vi "SVI_gauss_proba.vi"(4 "Delta":dbl, 5 "Seuil":dbl) -> (0 "Mu+ Delta":dbl, 1 "Mu-Delta":dbl, 2 "proba (Mu-Delta<X< Mu + Delta)":dbl(knob) scale=0.0..100.0, 3 "proba (X<Seuil)":dbl(knob) scale=0.0..100.0)   [LabVIEW 2010, in "lv_02.lvlib"]
uses:
  lv_02/p_5E1_LN.ctl
  lv_02/lv_02.lvlib
panel:
  in  "Paramètres Loi de Gauss":T1
  # "MODELE DE GAUSS\nF(Seuil)=prob(X<Seuil) \nprob (m-Delta<X<m+delta) \nsi X ---> N(m,sigma)"
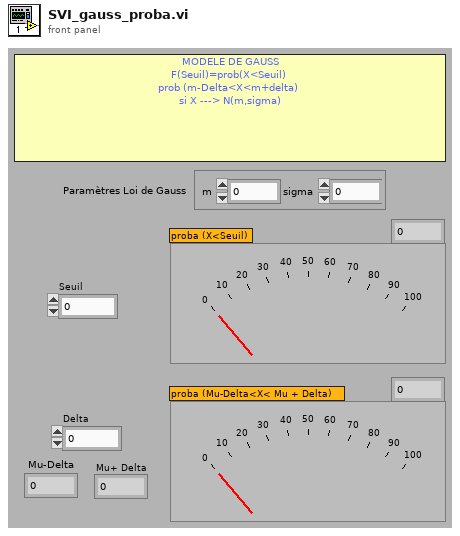
[diagram p1: front panel]
types:
  T1 = typedef "lv_02.lvlib/p_5E1_LN.ctl" = cluster{"m":dbl, "sigma":dbl}
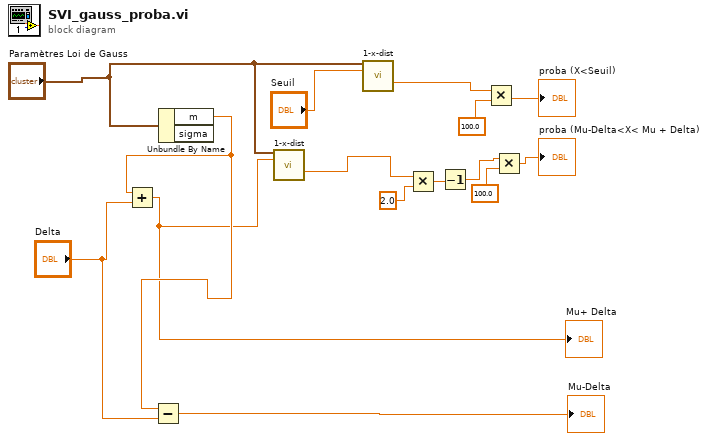
[diagram p0: block diagram]
diagram:
  n1 = Unbundle By Name("Paramètres Loi de Gauss") -> ("m"=w4:dbl)  [unwired: 1 out]
  n2 = Add(x=w4, y="Delta") -> (x+y=w2:dbl)
  "Mu+ Delta" <- w2
  n3 = Subtract(x=w4, y="Delta") -> (x-y=→"Mu-Delta":dbl)
  n4 = call "1-x-dist.vi"("p_LN"="Paramètres Loi de Gauss", "x"=w2) -> ("F(x)"=w3:dbl)  [unwired: 9 in, 4 out]
  n5 = call "1-x-dist.vi"("p_LN"="Paramètres Loi de Gauss", "x"="Seuil") -> ("F(x)"=w5:dbl)  [unwired: 9 in, 4 out]
  n6 = Multiply(x=w3, y=2.0) -> (x*y=w12:dbl)
  n7 = Decrement(x=w12) -> (x-1=w10:dbl)
  n8 = Multiply(x=w5, y=100.0) -> (x*y=→"proba (X<Seuil)":dbl)
  n9 = Multiply(x=w10, y=100.0) -> (x*y=→"proba (Mu-Delta<X< Mu + Delta)":dbl)
